vi "WPI_PWMSetValue.vi"(8 "error in (no error)":errorcluster, 9 "Value":u16, 11 "PWMDeviceRef":T1={"DeviceStatus"={"status"=FALSE, "code"=0, "source"=""}, "PWM Channel"=enum."PWM 1"}) -> (0 "error out":errorcluster, 3 "PWMDeviceRef":T1={"DeviceStatus"={"status"=FALSE, "code"=0, "source"=""}, "PWM Channel"=enum."PWM 1"})   [LabVIEW 2017]
doc: "Specifies the motion of the PWM using a PWM value from 0 to 255. The raw PWM value ranges from 0 to 255. A value of 1 puts the motor controller in full reverse, a value of 255 puts the motor controller in full forward, and a value of 0 disables the motor controller. Use this VI with custom motor controllers. Use the SetSpeed VI on the MotorControl palette to specify PWM values for the Jaguar or Victor motor controllers.\n\nThis software is licensed. Open the labview\\readme\\WPI Robotics Library Open Source License.txt file for more information."
uses:
  <vilib>/Rock Robotics/WPI/PWM/WPI_PWMDeviceRef.ctl
  <vilib>/Rock Robotics/SystemInterfaces/DIO/FPGA_DIOPWMChannel.ctl
  <vilib>/Rock Robotics/WPI/PWM/WPI_PWMChannelCacheOp.ctl
  <vilib>/Rock Robotics/WPI/PWM/WPI_PWMSafetyCheck.vi
  <instrlib>/Parallax Standard Servo/HAIOL/Parallax Standard Servo.lvclass
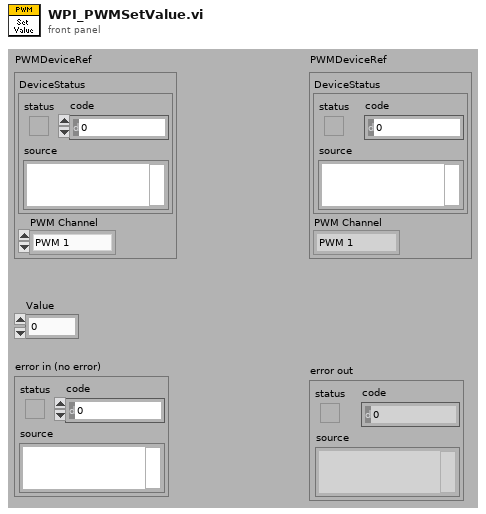
[diagram p1: front panel]
types:
  T1 = typedef "WPI_PWMDeviceRef.ctl" = cluster{"DeviceStatus":errorcluster, "PWM Channel":T2}
  T2 = typedef "FPGA_DIOPWMChannel.ctl" = enum8{"PWM 0", "PWM 1", "PWM 2", "PWM 3", "PWM 4", "PWM 5", "PWM 6", "PWM 7", "PWM 8", "PWM 9", "PWM MXP 0", "PWM MXP 1", "PWM MXP 2", "PWM MXP 3", "PWM MXP 4", "PWM MXP 5", "PWM MXP 6", "PWM MXP 7", "PWM MXP 8", "PWM MXP 9", "Invalid"}
  T3 = typedef "WPI_PWMChannelCacheOp.ctl" = enum16{"Acquire", "Release", "Status"}
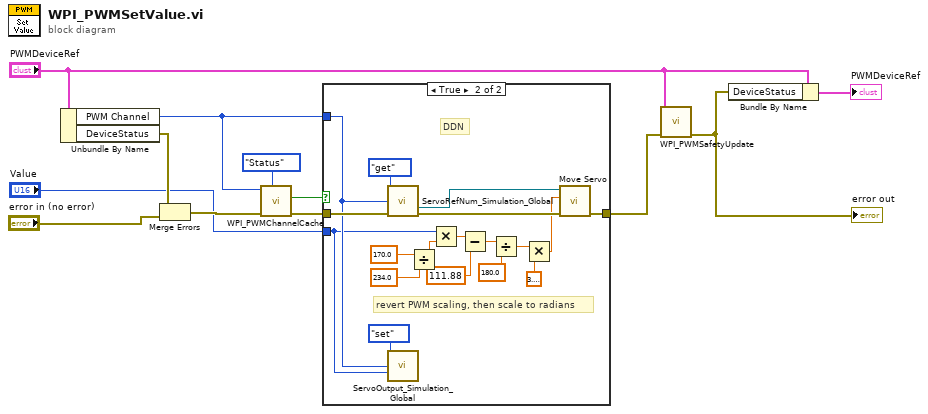
[diagram p0: block diagram]
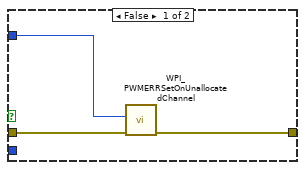
[diagram p2: hidden frame]
diagram:
  n1 = Unbundle By Name("PWMDeviceRef") -> ("PWM Channel"=w5:T2, "DeviceStatus"=w7:errorcluster)
  n2 = Merge Errors(w7, "error in (no error)") -> (w6:errorcluster)
  n3 = call <vilib>:"WPI_PWMChannelCache.vi"("Operation"=WPI_PWMChannelCacheOp."Status", "error in (no error)"=w6, "PWMChannel"=w5) -> ("error out"=w3:errorcluster, "Allocated?"=w4:bool)  [unwired: 2 in, 5 out]
  n4 = case shown="True" w4 {
    tunnel: w3 -> [w15 w32]
    tunnel: [w14 w29] -> w1
    tunnel: w5 -> [w13 w17]
    tunnel: "Value" -> [_ w16]
    frame False {
      n5 = call <vilib>:"WPI_PWMERRSetOnUnallocatedChannel.vi"("error in (no error)"=w15, "PWM Channel"=w13) -> ("error out"=w14:errorcluster)  [unwired: 9 in]
    }
    frame True {
      # "DDN"
      # "revert PWM scaling, then scale to radians"
      n6 = call <vilib>:"ServoRefNum_Simulation_Global.vi"("menu"=enum16{"set", "get", "delete"}."get", "PWM Channel"=w17, "error in (no error)"=w32) -> ("Servo Get"=w30:refnum<class "Parallax Standard Servo.lvclass">, "error out"=w31:errorcluster)  [unwired: 11 in]
      n7 = call <vilib>:"ServoOutput_Simulation_Global.vi"("menu"=enum16{"set", "get", "delete"}."set", "PWM Channel"=w17, "Output Set"=w16) -> ()  [unwired: 11 in, 2 out]
      n8 = Divide(x=170.0, y=234.0) -> (x/y=w26:dbl)
      n9 = Multiply(x=w16, y=w26) -> (x*y=w25:dbl)
      n10 = Subtract(x=w25, y=111.88) -> (x-y=w23:dbl)
      n11 = Divide(x=w23, y=180.0) -> (x/y=w20:dbl)
      n12 = Multiply(x=w20, y=3.141592653589793) -> (x*y=w21:dbl)
      n13 = call-dynamic "Move Servo.vi"("error in (no error)"=w31, "CCW Position (0.0 rad)"=w21, "Parallax Standard Servo in"=w30) -> ("error out"=w29:errorcluster)  [unwired: 7 in, 1 out]
    }
  }
  n14 = call <vilib>:"WPI_PWMSafetyUpdate.vi"("error in (no error)"=w1, "PWMDeviceRef"="PWMDeviceRef") -> ("error out"=w10:errorcluster)  [unwired: 9 out]
  "error out" <- w10
  n15 = Bundle By Name(cluster="PWMDeviceRef", "DeviceStatus"=w10) -> (→"PWMDeviceRef":T1)
